vi "OCT Reference Follower v1.3.vi"(6 "stop":bool, 7 "OCT Act ON":bool=TRUE, 8 "OCT Z PID Gains":cluster{"Kp":dbl, "Kd":dbl, "Ki":dbl}={"Kp"=0.0003, "Kd"=0.0001, "Ki"=0.01}, 9 "OCT  Z cmd Posit [mm]":dbl, 10 "error in":errorcluster, 11 "FPGA VI Reference In":refnum<k20>) -> (1 "OCT  Z out Posit [mm]":dbl, 2 "error out":errorcluster, 3 "FPGA VI Reference Out":refnum<k20>)   [LabVIEW 2010]
uses:
  <vilib>/rvi/interface/nirviReadWriteControl/nirviReadWriteControl.xnode
  Library/jmslib.lvlib
  FPGA Bitfiles/IRISSControl_FPGATarget_IRISSFPGAIOv3.3_r-h2UkgnQFc.lvbitx
  IRISS_FPGA_IO_v3.3.vi
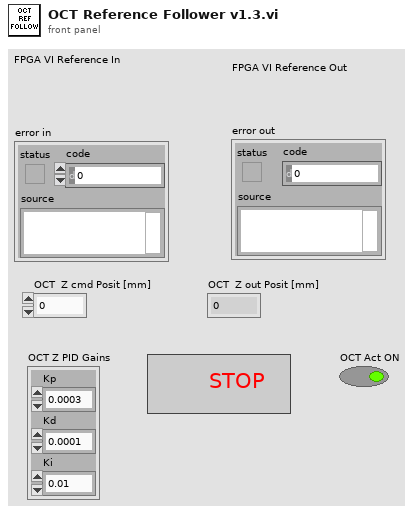
[diagram p1: front panel]
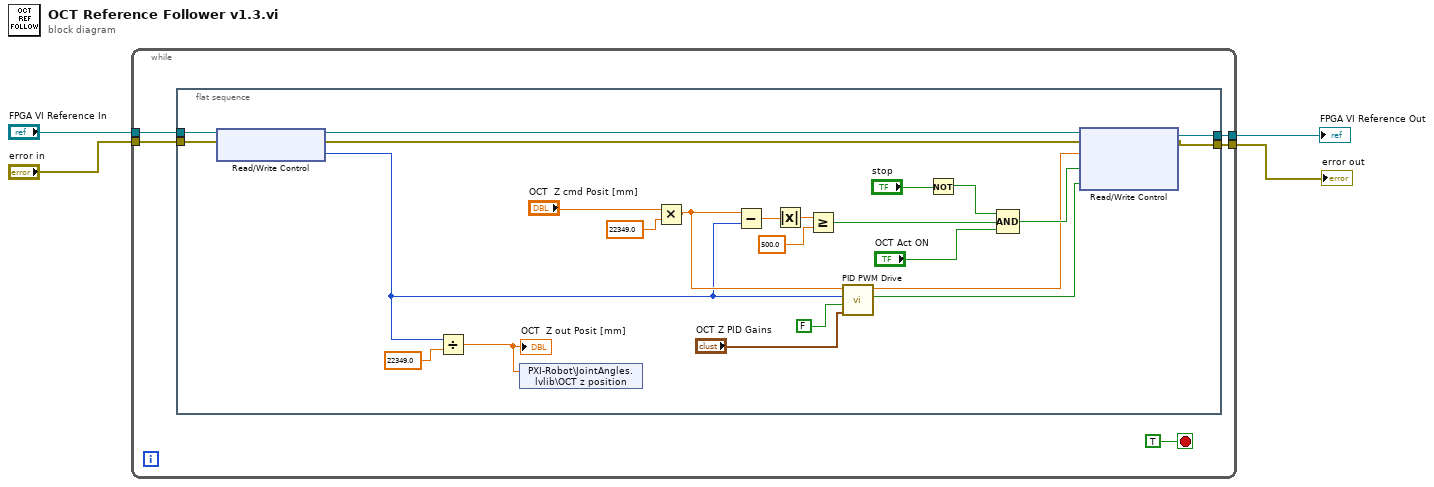
[diagram p0: block diagram]
diagram:
  n1 = while {
    tunnel: "FPGA VI Reference In" -> [w9]
    tunnel: "error in" -> [w8]
    tunnel: [w7] -> w4
    tunnel: [w6] -> w3
    stop <- TRUE stop-if-true
    n2 = flat-sequence {
      tunnel: w9 -> [w33]
      tunnel: w8 -> [w32]
      tunnel: [w31] -> w7
      tunnel: [w30] -> w6
      frame #0 {
        n3 = xnode "Read/Write Control"("FPGA VI Reference In"=w33, "error in"=w32) -> ("FPGA VI Reference Out"=w29:refnum<k20>, "error out"=w28:errorcluster, "32 bit Position 14"=w10:i32)
        n4 = Divide(x=w10, y=22349.0) -> (x/y=w11:dbl)
        "OCT  Z out Posit [mm]" <- w11
        n5 = shared-variable "PXI-Robot\\JointAngles.lvlib\\OCT z position"(w11) -> ()  [unwired: 1 in, 1 out]
        n6 = Multiply(x="OCT  Z cmd Posit [mm]", y=22349.0) -> (x*y=w22:dbl)
        n7 = Subtract(x=w22, y=w10) -> (x-y=w27:dbl)
        n8 = Absolute Value(x=w27) -> (abs(x)=w26:dbl)
        n9 = Greater Or Equal?(x=w26, y=500.0) -> (x >= y?=w17:bool)
        n10 = call "PID PWM Drive.vi"("PID Gains"="OCT Z PID Gains", "Reverse Motor?"=FALSE, "Encoder Position"=w10, "Reference"=w22) -> ("Direction"=w16:bool, "Duty Cycle"=w14:dbl)  [unwired: 5 in, 1 out]
        n11 = Not(x="stop") -> (.not. x?=w18:bool)
        n12 = Compound Arithmetic op=AND(w18, w17, "OCT Act ON") -> (w15:bool)
        n13 = xnode "Read/Write Control"("FPGA VI Reference In"=w29, "error in"=w28, "OCT Mot DC"=w14, "INHB OCT Mot"=w15, "DIR OCT Mot"=w16) -> ("FPGA VI Reference Out"=w31:refnum<k20>, "error out"=w30:errorcluster)
      }
    }
  }
  "error out" <- w3
  "FPGA VI Reference Out" <- w4
